vi "DoCreateError.vi"(5 "MergeErrors":bool, 6 "AdditionalText":string, 7 "Data":variant, 8 "ErrorIn":errorcluster caption="Error In", 9 "Text":string, 10 "ErrorCode":i32, 11 "ObjectIn":refnum<class "ErrorCreationTAF.lvclass"> caption="Object In") -> (0 "ErrorOut":errorcluster caption="Error Out", 3 "ObjectOut":refnum<class "ErrorCreationTAF.lvclass"> caption="Object Out")   [LabVIEW 2021, in "ErrorCreationTAF.lvclass"]
uses:
  ErrorCreationTAF.lvclass
  fec1759e-50a6-418f-9aeb-0391d960c39c.vi
  2053c0c2-6fc7-4aef-8a82-02155042cfc7.vi
  eaf0681e-e464-4b3a-95e7-fa23abfdab0d.vi
  7ef92f3e-c7f7-412d-a1f5-49b3e5bac52a.vi
  <vilib>/TriekselSoft/TracerLibrary/TracerLibrary/Tracer/protected/SendMessage.vi
  <vilib>/TriekselSoft/TracerLibrary/TracerLibrary/Tracer/protected/Timestamp.vi
  <vilib>/JDP Science/JSONtext/Variant to JSON Text.vi
  <vilib>/TriekselSoft/TracerLibrary/TracerLibrary/Tracer/Tracer_Level-Error.vi
  <vilib>/TriekselSoft/TracerLibrary/TracerLibrary/Tracer/protected/Tracer_ClassAttributes.vi
  <vilib>/JDP Science/JSONtext/LVClass Serializer/JSONtext LVClass Serializer.lvclass
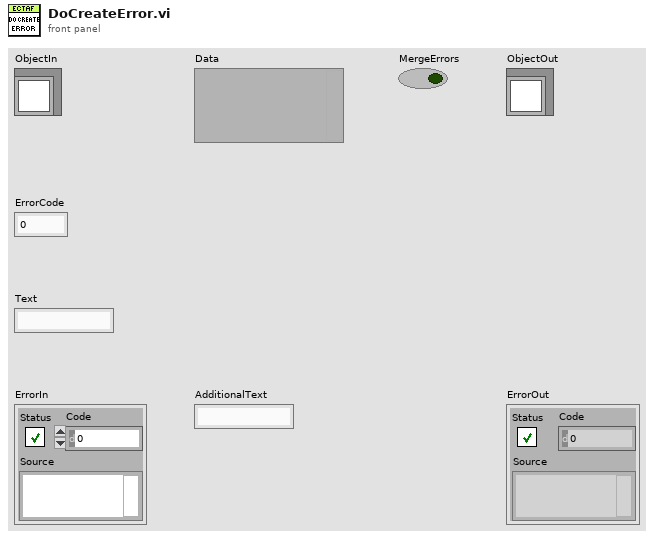
[diagram p1: front panel]
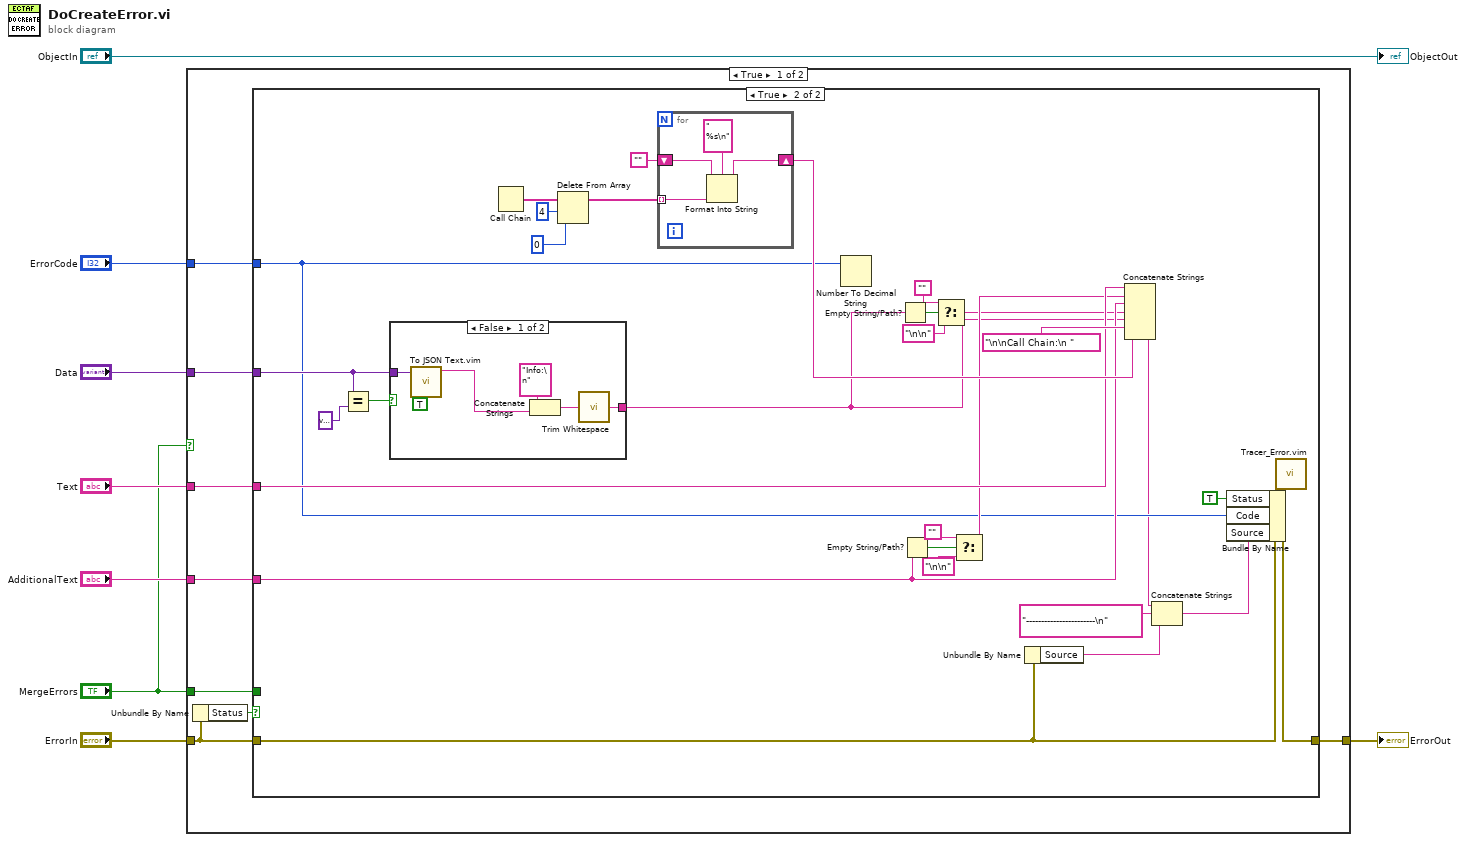
[diagram p0: block diagram]
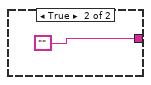
[diagram p3: hidden frame]
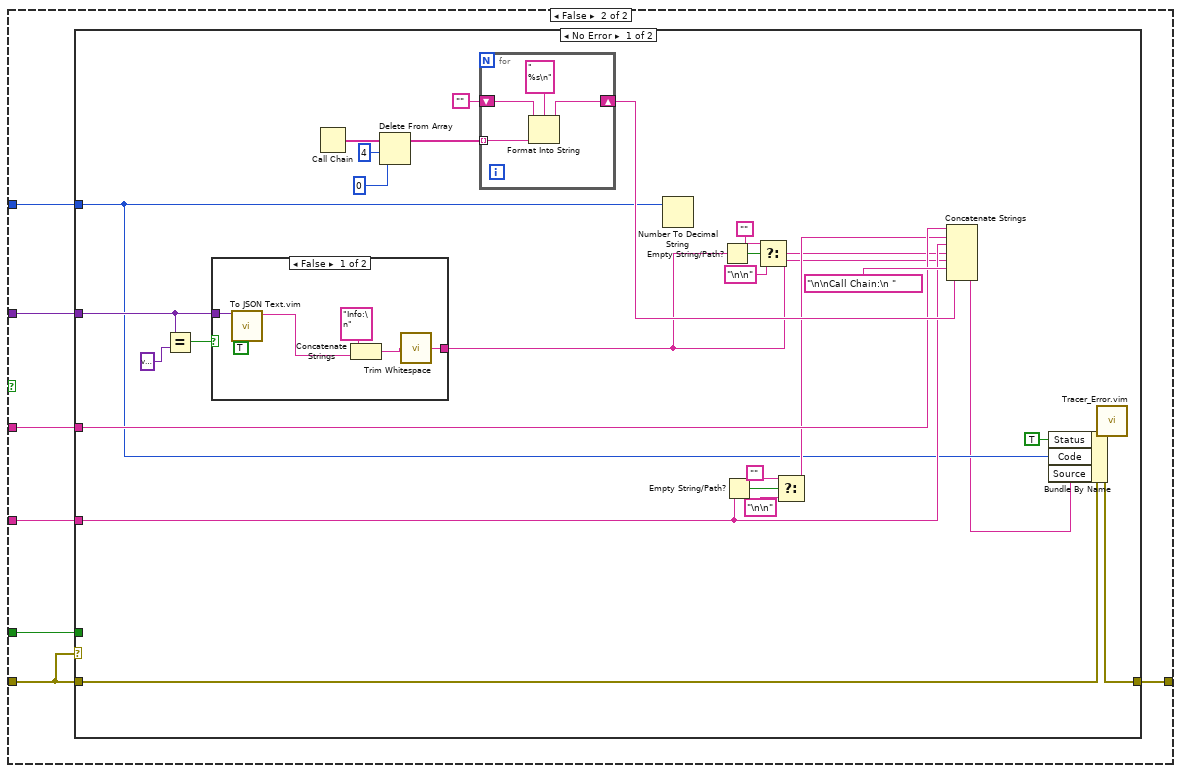
[diagram p4: hidden frame]
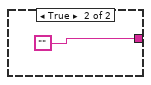
[diagram p5: hidden frame]
diagram:
  n1 = case shown="True" "MergeErrors" {
    tunnel: [w16 w64] -> w8
    tunnel: "Data" -> [w14 w62]
    tunnel: "Text" -> [w13 w61]
    tunnel: "AdditionalText" -> [w12 w60]
    tunnel: "ErrorCode" -> [w11 w59]
    tunnel: "MergeErrors" -> [w10 w58]
    tunnel: "ErrorIn" -> [w15 w63]
    frame True {
      n2 = Unbundle By Name(w15) -> ("Status"=w9:bool)
      n3 = case shown="True" w9 {
        tunnel: w15 -> [w17 w46]
        tunnel: [w17 w18] -> w16
        tunnel: w14 -> [_ w45]
        tunnel: w13 -> [_ w34]
        tunnel: w12 -> [_ w28]
        tunnel: w11 -> [_ w23]
        tunnel: w10 -> [_ _]
        frame False {
        }
        frame True {
          n4 = Equal?(x=w45, y=variant) -> (x = y?=w42:bool)
          n5 = case shown="False" w42 {
            tunnel: [w54 ""] -> w26
            tunnel: w45 -> [w53 _]
            frame False {
              n6 = call "To JSON Text.vim"("Pretty Print?"=TRUE, "Anything"=w53) -> ("<JSON>"=w51:string)  [unwired: 8 in, 1 out]
              n7 = Concatenate Strings("Info:\n" ("string"), w51) -> (w56:string)
              n8 = call <vilib>:"Trim Whitespace.vi"("string"=w56) -> ("trimmed string"=w54:string)  [unwired: 1 in]
            }
            frame True {
            }
          }
          n9 = Call Chain() -> (call chain=w40:string[])
          n10 = Delete From Array(array=w40, length=4, index=0 ("length")) -> (array with subset deleted=w39:string[])  [unwired: 1 out]
          n11 = for {
            tunnel: w39 -> [w50] mode=indexing
            shift-right: [w48] -> w35
            shift-left: "" -> [w49]
            n12 = Format Into String(format string="  %s\n", initial string=w49, w50) -> (resulting string=w48:string)  [unwired: 1 in, 1 out]
          }
          n13 = Number To Decimal String(number=w23) -> ()  [unwired: 1 in, 1 out]
          n14 = Empty String/Path?(string/path=w26) -> (empty?=w30:bool)
          n15 = Empty String/Path?(string/path=w28) -> (empty?=w33:bool)
          n16 = Select(t="", s=w30, f="\n\n") -> (s? t:f=w27:string)
          n17 = Select(t="", s=w33, f="\n\n") -> (s? t:f=w29:string)
          n18 = Unbundle By Name(w46) -> ("Source"=w22:string)
          n19 = Concatenate Strings(w34, w29, w28, w27, w26, "\n\nCall Chain:\n " ("format string"), w35) -> (w20:string)
          n20 = Concatenate Strings(w20, "-----------------------\n" ("string"), w22) -> (w19:string)
          n21 = Bundle By Name(cluster=w46, "Status"=TRUE ("status"), "Code"=w23, "Source"=w19) -> (w18:errorcluster)
          n22 = call "Tracer_Error.vim"("Error In"=w18) -> ()  [unwired: 10 in, 1 out]
        }
      }
    }
    frame False {
      n23 = case shown="No Error" w63 {
        tunnel: w63 -> [w90 w102]
        tunnel: [w65 w102] -> w64
        tunnel: w62 -> [w89 _]
        tunnel: w61 -> [w78 _]
        tunnel: w60 -> [w72 _]
        tunnel: w59 -> [w67 _]
        tunnel: w58 -> [_ _]
        frame No Error {
          n24 = Equal?(x=w89, y=variant) -> (x = y?=w86:bool)
          n25 = case shown="False" w86 {
            tunnel: [w100 ""] -> w70
            tunnel: w89 -> [w96 _]
            frame False {
              n26 = call "To JSON Text.vim"("Pretty Print?"=TRUE, "Anything"=w96) -> ("<JSON>"=w97:string)  [unwired: 8 in, 1 out]
              n27 = Concatenate Strings("Info:\n" ("string"), w97) -> (w95:string)
              n28 = call <vilib>:"Trim Whitespace.vi"("string"=w95) -> ("trimmed string"=w100:string)  [unwired: 1 in]
            }
            frame True {
            }
          }
          n29 = Call Chain() -> (call chain=w84:string[])
          n30 = Delete From Array(array=w84, length=4, index=0 ("length")) -> (array with subset deleted=w83:string[])  [unwired: 1 out]
          n31 = for {
            tunnel: w83 -> [w94] mode=indexing
            shift-right: [w92] -> w79
            shift-left: "" -> [w93]
            n32 = Format Into String(format string="  %s\n", initial string=w93, w94) -> (resulting string=w92:string)  [unwired: 1 in, 1 out]
          }
          n33 = Number To Decimal String(number=w67) -> ()  [unwired: 1 in, 1 out]
          n34 = Empty String/Path?(string/path=w70) -> (empty?=w74:bool)
          n35 = Empty String/Path?(string/path=w72) -> (empty?=w77:bool)
          n36 = Select(t="", s=w74, f="\n\n") -> (s? t:f=w71:string)
          n37 = Select(t="", s=w77, f="\n\n") -> (s? t:f=w73:string)
          n38 = Concatenate Strings(w78, w73, w72, w71, w70, "\n\nCall Chain:\n " ("format string"), w79) -> (w66:string)
          n39 = Bundle By Name(cluster=w90, "Status"=TRUE ("status"), "Code"=w67, "Source"=w66) -> (w65:errorcluster)
          n40 = call "Tracer_Error.vim"("Error In"=w65) -> ()  [unwired: 10 in, 1 out]
        }
        frame Error {
        }
      }
    }
  }
  "ErrorOut" <- w8
  "ObjectOut" <- "ObjectIn"
